vi "Create Coverage Analyzer View.vi"(8 "error in (no error)":errorcluster, 10 "Code Coverage":map{path, dbl}(c390)) -> (0 "error out":errorcluster, 3 "Coverage Analyzer Result View out":refnum<class "Coverage Analyzer Result View.lvclass">)   [LabVIEW 2020, in "Coverage Analyzer.lvlib" / "Coverage Analyzer Result View.lvclass"]
uses:
  Coverage Analyzer Result View.lvclass
  Coverage Analyzer Result View.lvclass/Coverage Analyzer Result View.ctl
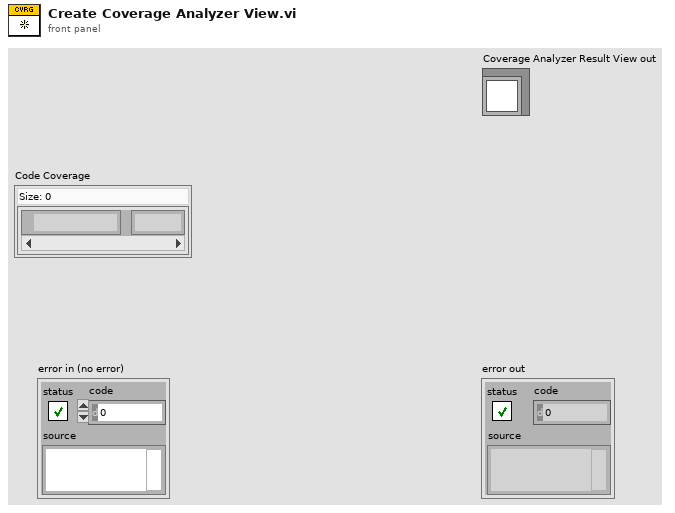
[diagram p1: front panel]
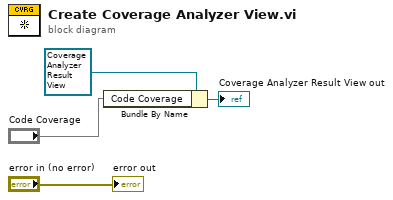
[diagram p0: block diagram]
diagram:
  n1 = Bundle By Name(cluster=refnum<class "Coverage Analyzer Result View.lvclass"> refnum ("Coverage Analyzer Result View.lvclass"), "Code Coverage"="Code Coverage") -> (→"Coverage Analyzer Result View out":refnum<class "Coverage Analyzer Result View.lvclass">)
  "error out" <- "error in (no error)"
